vi "get source path start.vi"(0 "main VI path":path) -> (4 "source file path":path)   [LabVIEW 2019]
doc: "This subVI uses the main VI's path as a reference pointer to choose the source data file path."
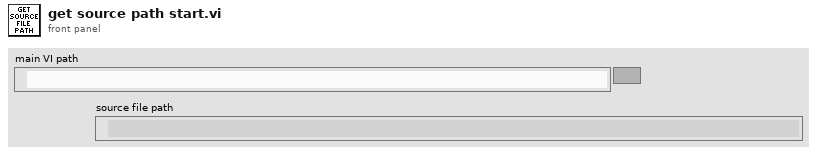
[diagram p1: front panel]
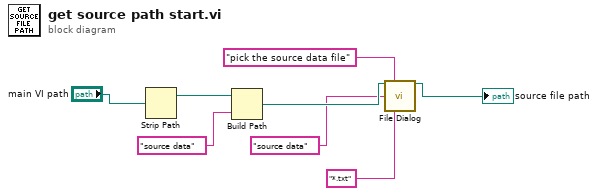
[diagram p0: block diagram]
diagram:
  n1 = Strip Path(path="main VI path") -> (stripped path=w7:path)  [unwired: 1 out]
  n2 = Build Path(base path=w7, name or relative path="source data") -> (appended path=w4:path)
  n3 = call "File Dialog"("start path"=w4, "prompt"="pick the source data file", "default name"="source data", "pattern (all files)"="*.txt") -> ("selected path"=→"source file path":path)  [unwired: 8 in, 3 out]
